vi "RewireDynamicDispatchTerminals.vi"(8 "error in (no error)":errorcluster, 10 "VI Reference":refnum<vi>, 11 "LVClassLibrary":refnum<vi>) -> (0 "error out":errorcluster, 2 "VI Reference":refnum<vi>, 3 "LVClassLibrary":refnum<vi>)   [LabVIEW 2019, in "BlueSerializationScripts.lvlib"]
uses:
  BlueSerializationScripts.lvlib
  NI_Branches/BlueBranch_CLSUIP.lvlib
  BlueUtilityScripts/BlueUtilityScripts.lvlib
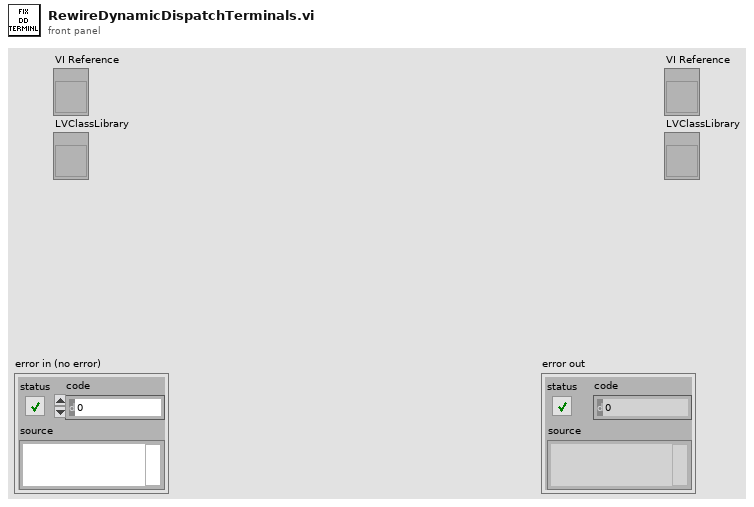
[diagram p1: front panel]
types:
  T1 = enum16{"Invalid Wire Rule", "Required", "Recommended", "Optional", "Dynamic Dispatch"}
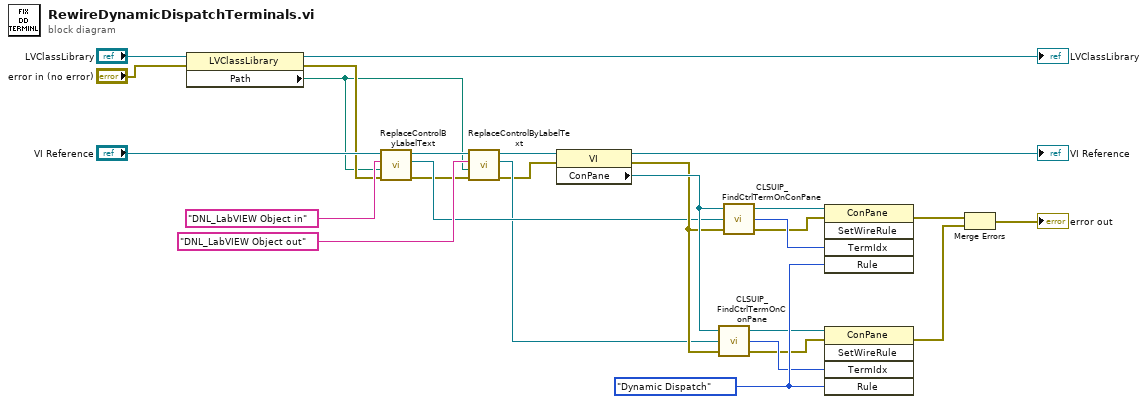
[diagram p0: block diagram]
diagram:
  w27 = T1."Dynamic Dispatch" ("Rule")
  n1 = property class="LVClassLibrary"(reference="LVClassLibrary", error in="error in (no error)") -> (reference out=→"LVClassLibrary":refnum<vi>, error out=w4:errorcluster, "Path"=w2:path)
  n2 = call "ReplaceControlByLabelText.vi"("error in (no error)"=w4, "Replacement Path"=w2, "Control Label.text"="DNL_LabVIEW Object in" ("name"), "VI ref"="VI Reference") -> ("error out"=w3:errorcluster, "New Control Ref"=w7:refnum<vi>, "VI ref"=w9:refnum<vi>)  [unwired: 5 in]
  n3 = call "ReplaceControlByLabelText.vi"("error in (no error)"=w3, "Replacement Path"=w2, "Control Label.text"="DNL_LabVIEW Object out" ("name"), "VI ref"=w9) -> ("error out"=w1:errorcluster, "New Control Ref"=w6:refnum<vi>, "VI ref"=w5:refnum<vi>)  [unwired: 5 in]
  n4 = property class="VI"(reference=w5, error in=w1) -> (reference out=→"VI Reference":refnum<vi>, error out=w19:errorcluster, "ConPane"=w22:refnum<vi>)
  n5 = call "CLSUIP_FindCtrlTermOnConPane.vi"("error in (no error)"=w19, "Ctl Refnum"=w6, "ConPane"=w22) -> ("error out"=w17:errorcluster, "Terminal Index"=w20:i32, "ConPane out"=w21:refnum<vi>)
  n6 = call "CLSUIP_FindCtrlTermOnConPane.vi"("error in (no error)"=w19, "Ctl Refnum"=w7, "ConPane"=w22) -> ("error out"=w18:errorcluster, "Terminal Index"=w23:i32, "ConPane out"=w24:refnum<vi>)
  n7 = invoke class="ConPane" method="SetWireRule"(reference=w24, error in=w18, "TermIdx"=w23, "Rule"=w27) -> (error out=w26:errorcluster)  [unwired: 1 in, 4 out]
  n8 = invoke class="ConPane" method="SetWireRule"(reference=w21, error in=w17, "TermIdx"=w20, "Rule"=w27) -> (error out=w25:errorcluster)  [unwired: 1 in, 4 out]
  n9 = Merge Errors(w26, w25) -> (→"error out":errorcluster)
